vi "ATS_About.vi"(4 "NO Display":bool, 6 "Scrollbar Visible":bool, 7 "AboutIn":string) -> (2 "AboutOut":string="ATScope Version 6.0.8\nCopyright (C) 2003-2012\n\n" caption="About", 3 "Version#":string=" 4.8.2")   [LabVIEW 2010]
doc: "_____AlazarTech, Scope_____\n\nDisplay the ABOUT information until the OK button is activate unless NoDIsplay input is True then only the Version# output is read.\nIf Scrollbar is true a scrollbar will be display so the user can scroll on the text."
panel:
  in  "OK":bool
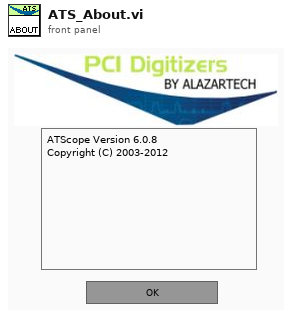
[diagram p1: front panel]
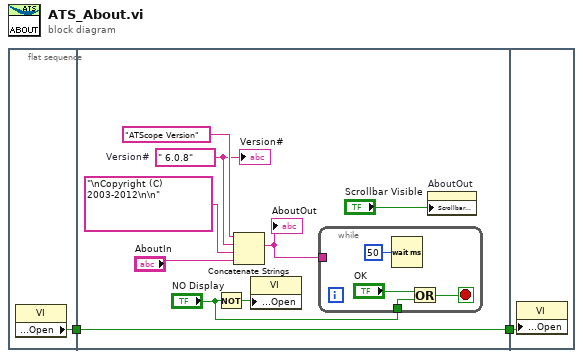
[diagram p0: block diagram]
diagram:
  n1 = flat-sequence {
    tunnel: [w3] -> w1
    tunnel: [w4] -> w2
    tunnel: w1 -> [w4]
    tunnel: w2 -> [w17]
    frame #0 {
      n2 = property class="VI"() -> ("Front Panel Window:Open"=w3:bool)  [unwired: 2 in, 2 out]
    }
    frame #1 {
      w7 = " 6.0.8"  # Version#
      n3 = Not(x="NO Display") -> (.not. x?=w6:bool)
      n4 = Concatenate Strings("ATScope Version" ("About"), w7, "\nCopyright (C) 2003-2012\n\n" ("About"), "AboutIn") -> (w10:string)
      "AboutOut" <- w10
      n5 = property class="VI"("Front Panel Window:Open"=w6) -> ()  [unwired: 2 in, 2 out]
      n6 = while {
        tunnel: w10 -> [_]
        tunnel: "NO Display" -> [w13]
        stop <- w14 stop-if-true
        n7 = Wait (ms)(milliseconds to wait=u32 50) -> ()  [unwired: 1 out]
        n8 = Or(x="OK", y=w13) -> (x .or. y?=w14:bool)
      }
      n9 = property on="AboutOut" class="Str"("Scrollbar Visible"="Scrollbar Visible") -> ()  [unwired: 2 in, 2 out]
      "Version#" <- w7
    }
    frame #2 {
      n10 = property class="VI"("Front Panel Window:Open"=w17) -> ()  [unwired: 2 in, 2 out]
    }
  }
